vi "Test Get Named Range Values (VAR).vi"(11 "Test Case In":refnum<class "Test Open Xml.lvclass">) -> (0 "error out":errorcluster, 3 "Test Case Out":refnum<class "Test Open Xml.lvclass">)   [LabVIEW 2020, in "Test Open Xml.lvclass"]
uses:
  Test Open Xml.lvclass
  e7d09ce7-04db-40ce-9c4e-a78b31ec9fe8.vi
  Source/Open Xml.lvlib
  50f757ab-2d74-46a0-bdd7-e6f0543e2c81.vi
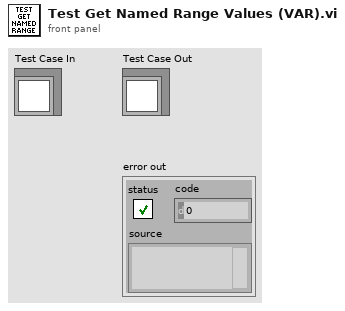
[diagram p1: front panel]
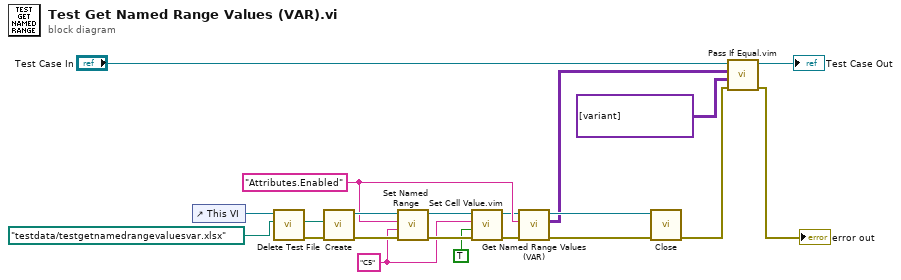
[diagram p0: block diagram]
diagram:
  w1 = "C5" ("Cell Address")
  w6 = "Attributes.Enabled" ("Sheet Name")
  n1 = control-ref of="This VI"() -> (w11:refnum<vi>)
  n2 = call "Delete Test File.vi"("name or relative path"=path "testdata/testgetnamedrangevaluesvar.xlsx", "VI in"=w11) -> ("error out"=w9:errorcluster, "deleted path"=w10:path)  [unwired: 8 in]
  n3 = call "Create.vi"("error in"=w9, "Path"=w10) -> ("error out"=w18:errorcluster, "SpreadsheetDoc"=w7:refnum<k24>)  [unwired: 8 in]
  n4 = call "Set Named Range.vi"("error in"=w18, "Cell Range"=w1, "Named Range Identifier"=w6, "SpreadsheetDoc in"=w7) -> ("error out"=w8:errorcluster, "SpreadsheetDoc out"=w4:refnum<k24>)  [unwired: 6 in]
  n5 = call "Set Cell Value.vim"("error in"=w8, "Value"=TRUE, "Cell Address"=w1, "SpreadsheetDoc in"=w4) -> ("error out"=w5:errorcluster, "SpreadsheetDoc out"=w3:refnum<k24>)  [unwired: 6 in]
  n6 = call "Get Named Range Values (VAR).vi"("error in"=w5, "Named Range Identifier"=w6, "SpreadsheetDoc in"=w3) -> ("error out"=w17:errorcluster, "Cells"=w14:variant[][], "SpreadsheetDoc out"=w15:refnum<k24>)  [unwired: 6 in]
  n7 = call "Close.vi"("error in"=w17, "SpreadsheetDoc"=w15) -> ("error out"=w16:errorcluster)  [unwired: 9 in]
  n8 = call "Pass If Equal.vim"("error in (no error)"=w16, "Actual"=variant[][] [[variant(bool TRUE)]] ("Cells"), "Expected"=w14, "LUnit Test Case In"="Test Case In") -> ("error out"=→"error out":errorcluster, "LUnit Test Case Out"=→"Test Case Out":refnum<class "Test Open Xml.lvclass">)  [unwired: 6 in]
